vi "Create logger.vi"(7 "LogLevel":T2, 8 "error in (no error)":errorcluster, 10 "UI Config":T1={"BG Color"=16448250, "Text Color"=3421236, "Font Size"=18, "Bold?"=TRUE}, 11 "Text File Configuration":T3={"Folder"=path "C:/Temp/CANLOG", "Name"="CAN_LOG", "Extension"="txt", "Max Size (MB)"=3, "Timestamp Filename"=TRUE}) -> (0 "error out":errorcluster)   [LabVIEW 2020]
uses:
  composed-event-logger/Source/Text File Sink/Configuration.ctl
  composed-event-logger/Source/Composed Log/Types/Log Level.ctl
  composed-event-logger/Source/ConsoleView/View/TypeDef/String Config.ctl
  composed-event-logger/Source/Composed Log/Log Sink/Sink Error Actions ENUM.ctl
  composed-event-logger/Source/Composed Log/LoggerReference/LoggerReference.lvclass/LoggerReference.ctl
  18945a94-c8f6-4ab5-b013-52b2f19072e1.vi
  18945a94-c8f6-4ab5-b013-52b2f19072e1.vi/c2ca87a3-4f6c-4c67-af72-aa7645b82f15.vi
  composed-event-logger/Source/Composed Log/LoggerReference/Return Aggregate Queues.vi
  composed-event-logger/Source/Composed Log/LoggerReference/Add Aggregate Log.vi
  18945a94-c8f6-4ab5-b013-52b2f19072e1.vi/c2ca87a3-4f6c-4c67-af72-aa7645b82f15.vi/554874db-e9cf-45d4-81c2-1db3cd36d289.vi
  composed-event-logger/Source/Composed Log/LoggerReference/Send Add Sink.vi
  composed-event-logger/Source/Text File Sink/Text File Sink.lvclass
  D:/Git/JabilTestLib/composed-event-logger/Source/Composed Log/Log Sink/Log Sink.lvclass
  composed-event-logger/Source/ConsoleView/Sink/ConsoleSink.lvclass
  global variable.vi
  composed-event-logger/Source/Composed Log/Application Logger/Launch Worker Loop.vi
  composed-event-logger/Source/Composed Log/LoggerReference/Initialize Logger Instance.vi
  composed-event-logger/Source/Composed Log/Singleton Event Log/Logger Queue FGV.vi
  composed-event-logger/Source/Composed Log/IErrorFormat/IErrorFormat.lvclass
  composed-event-logger/Source/Composed Log/LoggerReference/LoggerReference.lvclass
  composed-event-logger/Source/Composed Log/Log Sink/Log Sink.lvclass
  composed-event-logger/Source/ConsoleView/ConsoleInterface/ConsoleSession.lvclass
  composed-event-logger/Source/Composed Log/Composed Log.lvlib
  composed-event-logger/Source/ConsoleView/View/ConsoleView.lvclass
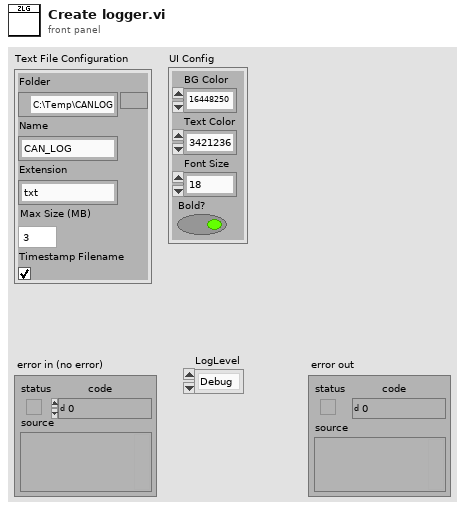
[diagram p1: front panel]
types:
  T1 = typedef "ConsoleView.lvlib/ConsoleView.lvclass/String Config.ctl" = cluster{"BG Color":u32, "Text Color":u32, "Font Size":u32, "Bold?":bool}
  T2 = typedef "Composed Log.lvlib/Log Level.ctl" = enum16{"Debug", "Info", "Warning", "Error", "Critical"}
  T3 = typedef "Text File Sink.lvclass/Configuration.ctl" = cluster{"Folder":path, "Name":string, "Extension":string, "Max Size (MB)":i64, "Timestamp Filename":bool}
  T4 = typedef "Composed Log.lvlib/Log Sink.lvclass/Sink Error Actions ENUM.ctl" = enum16{"Ignore Error and Continue", "Ignore Error and Close Sink", "Report Error and Close Sink"}
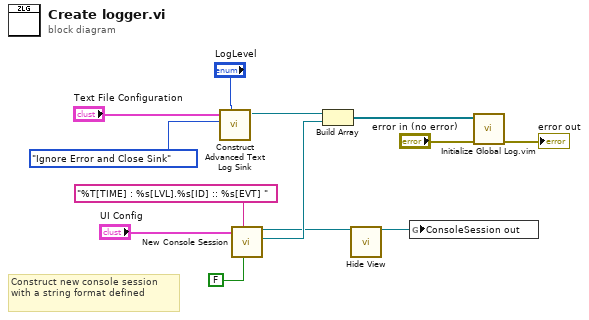
[diagram p0: block diagram]
diagram:
  # "Construct new console session with a string format defined"
  n1 = call "Construct Advanced Text Log Sink.vi"("LogLevel"="LogLevel", "Error Action"=Sink_Error_Actions_ENUM."Ignore Error and Close Sink", "Text File Configuration"="Text File Configuration") -> ("Text File Sink out"=w5:refnum<class "Text File Sink.lvclass">)  [unwired: 8 in]
  n2 = call "New Console Session.vi"("Persist After Shutdown?(F)"=FALSE, "Format Specifier"="%T[TIME] : %s[LVL].%s[ID] :: %s[EVT] ", "UI Config"="UI Config") -> ("ConsoleSink out"=w11:refnum<class "ConsoleSink.lvclass">, "ConsoleSession out"=w2:refnum<class "ConsoleSession.lvclass">)  [unwired: 6 in, 1 out]
  n3 = Build Array(w5, w11) -> (w13:refnum<class "Log Sink.lvclass">[])
  n4 = call "Hide View.vi"("ConsoleInterface in"=w2) -> ("ConsoleInterface out"=w1:refnum<class "ConsoleSession.lvclass">)  [unwired: 9 in, 1 out]
  n5 = global write "global variable.vi" "ConsoleSession out"(w1) -> ()
  n6 = call "Initialize Global Log.vim"("error in (no error)"="error in (no error)", "Log Sink(s)"=w13) -> ("error out"=→"error out":errorcluster)  [unwired: 8 in, 1 out]
